vi "AudioTest.Parse SoundCheck Results File.vi"(7 "SoundCheck Mic Data Name":string, 8 "error in":errorcluster, 9 "Primary Search String":string, 10 "Config Dir":path=path "C:/MTE/Audio Test/Config", 11 "Results Folder":path) -> (0 "error out":errorcluster, 1 "Name Lookup":variant, 2 "Mic":dbl, 3 "Meas":T1[](array[typedef]) {"Status" items=["LOG", "PASS", "FAIL", "ERROR"]}, 4 "Lookup File":path)   [LabVIEW 2018]
uses:
  Common/Utils/Results/Result.Measurement Item.ctl
  Common/Utils/Results/Result.Measurement and Attribute Item Status.ctl
panel:
  out "Data":string[][](array[string])
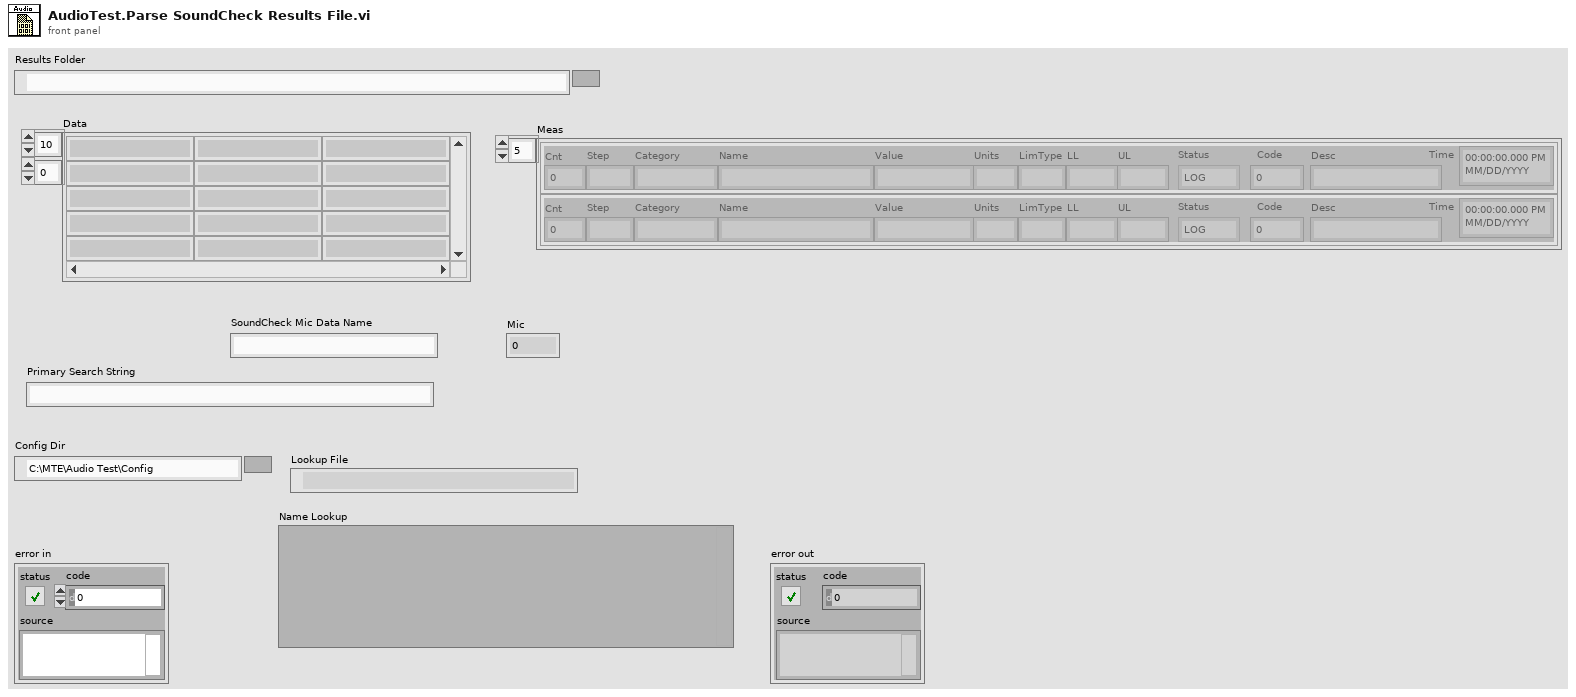
[diagram p1: front panel]
types:
  T1 = typedef "Result.Measurement Item.ctl" = cluster{"Cnt":i32, "Step":string, "Category":string, "Name":string, "Value":string, "Units":string, "LimType":string, "LL":string, "UL":string, "Status":T2, "Code":i32, "Desc":string, "Time":timestamp}
  T2 = typedef "Result.Measurement and Attribute Item Status.ctl" = i32
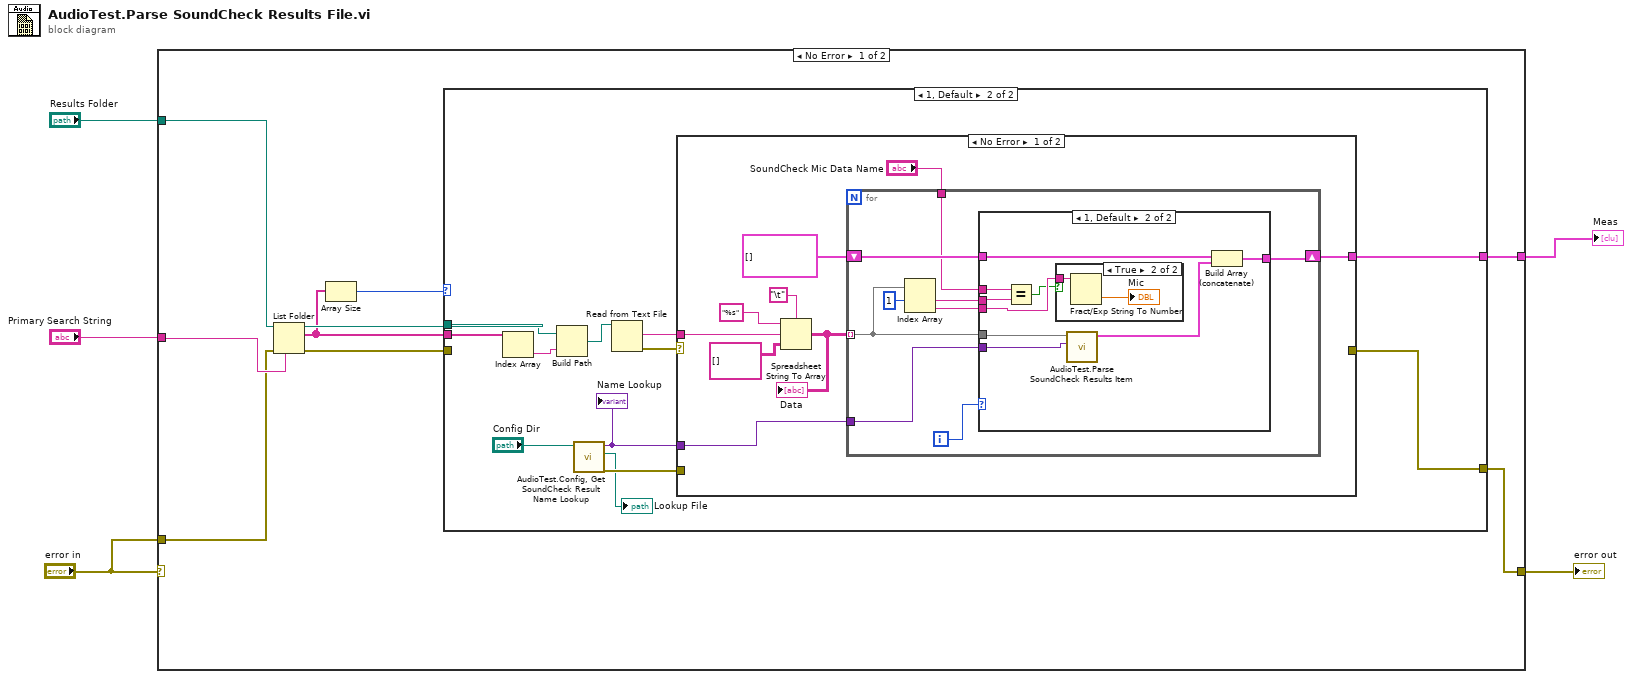
[diagram p0: block diagram]
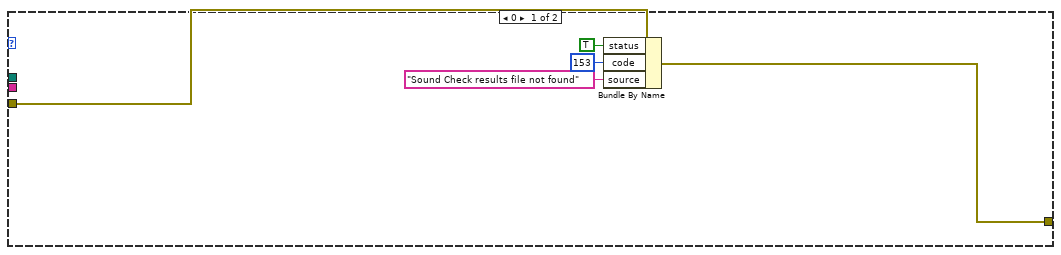
[diagram p2: hidden frame]
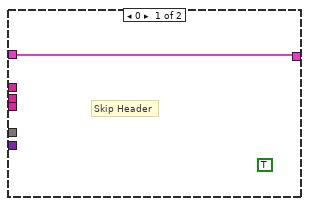
[diagram p3: hidden frame]
diagram:
  n1 = case shown="No Error" "error in" {
    selector: "error in" -> [_ w63]
    tunnel: "Results Folder" -> [w14 _]
    tunnel: [w13 w63] -> w4
    tunnel: [w12 _] -> w3
    tunnel: "Primary Search String" -> [w11 _]
    tunnel: "error in" -> [w10 _]
    frame No Error {
      n2 = List Folder(path=w14, pattern=w11, error in=w10) -> (path out=w8:path, filenames=w7:string[], error out=w6:errorcluster)  [unwired: 1 in, 1 out]
      n3 = Array Size(array=w7) -> (size(s)=w9:i32)
      n4 = case shown="1, Default" w9 {
        tunnel: w7 -> [_ w31]
        tunnel: w8 -> [_ w29]
        tunnel: [w18 w25] -> w13
        tunnel: [_ w24] -> w12
        tunnel: w6 -> [w19 _]
        frame 0 {
          n5 = Bundle By Name(cluster=w19, "status"=TRUE, "code"=153, "source"="Sound Check results file not found") -> (w18:errorcluster)
        }
        frame 1, Default {
          n6 = Index Array(array=w31) -> (element=w30:string)  [unwired: 1 in]
          n7 = Build Path(base path=w29, name or relative path=w30) -> (appended path=w28:path)
          n8 = call "AudioTest.Config, Get SoundCheck Result Name Lookup.vi"("Config Folder"="Config Dir") -> ("error out"=w21:errorcluster, "Lookup File"=→"Lookup File":path, "Name Lookup"=w22:variant)  [unwired: 8 in]
          "Name Lookup" <- w22
          n9 = Read from Text File(file (use dialog)=w28) -> (text=w27:string, error out=w26:errorcluster)  [unwired: 3 in, 2 out]
          n10 = case shown="No Error" w26 {
            selector: w26 -> [_ w62]
            tunnel: w27 -> [w40 _]
            tunnel: [_ w62] -> w25
            tunnel: [w35 _] -> w24
            tunnel: w22 -> [w33 _]
            tunnel: w21 -> [_ _]
            frame No Error {
              n11 = Spreadsheet String To Array(delimiter (Tab)="\t", format string="%s", spreadsheet string=w40, array type (2D Dbl)=string[][] []) -> (array=w34:string[][])
              "Data" <- w34
              n12 = for {
                tunnel: w34 -> [w45] mode=indexing
                shift-right: [w47] -> w35
                shift-left: T1[] [] ("Attributes") -> [w48]
                tunnel: w33 -> [w46]
                tunnel: "SoundCheck Mic Data Name" -> [w41]
                i -> [w49]
                n13 = Index Array(array=w45, index #1=1 ("index")) -> (element #1=w43:string, element #2=w42:string)  [unwired: 1 in]
                n14 = case shown="1, Default" w49 {
                  tunnel: w45 -> [_ w59]
                  tunnel: w48 -> [w50 w58]
                  tunnel: [w50 w57] -> w47
                  tunnel: w46 -> [_ w55]
                  tunnel: w43 -> [_ w54]
                  tunnel: w42 -> [_ w52]
                  tunnel: w41 -> [_ w53]
                  frame 0 {
                    (unwired) TRUE
                    # "Skip Header"
                  }
                  frame 1, Default {
                    n15 = Equal?(x=w53, y=w54) -> (x = y?=w51:bool)
                    n16 = case shown="True" w51 {
                      tunnel: w52 -> [_ w61]
                      frame False {
                      }
                      frame True {
                        n17 = Fract/Exp String To Number(string=w61) -> (number=→"Mic":dbl)  [unwired: 3 in, 1 out]
                      }
                    }
                    n18 = call "AudioTest.Parse SoundCheck Results Item.vi"("Name Lookup"=w55, "Result Record"=w59) -> ("Measurements"=w56:T1[])  [unwired: 9 in]
                    n19 = Build Array (concatenate)(w58, w56) -> (w57:T1[])
                  }
                }
              }
            }
            frame Error {
            }
          }
        }
      }
    }
    frame Error {
    }
  }
  "error out" <- w4
  "Meas" <- w3
